vi "Mouse Up on Plot.vi"(7 "Loop data in":T1={"TitleCollapse"=refnum, "MouseDownState"=enum."Idle", "RightClickCache"={"Mod"={"Ctrl"=FALSE, "Shift"=FALSE}, "CoordsStart"={"Horizontal"=0, "Vertical"=0}, "CoordsEnd"={"Horizontal"=0, "Vertical"=0}, "PlotAreaBounds"={"Left"=10, "Top"=10, "Right"=0, "Bottom"=0}, "slice"=[]}, "ZoomCache"={"SuppressedPlots"=[], "LeftAxis"={"NeedsRevert?"=FALSE, "Scale Fit"=0, "Range"={"Minimum"=0.0, "Maximum"=0.0, "Increment"=0.0, "Minor Increment"=0.0, "Start"=0.0}}, "RightAxis"={"NeedsRevert?"=FALSE, "Scale Fit"=0, "Range"={"Minimum"=0.0, "Maximum"=0.0, "Increment"=0.0, "Minor Increment"=0.0, "Start"=0.0}}, "Mod"={"Shift"=FALSE}}, "UpdateTime"=0.0, "keyboard"=refnum, "visible?"=FALSE}, 8 "error in (no error)":errorcluster, 11 "Refs":T12) -> (0 "error out":errorcluster, 5 "Loop data out":T1={"TitleCollapse"=refnum, "MouseDownState"=enum."Idle", "RightClickCache"={"Mod"={"Ctrl"=FALSE, "Shift"=FALSE}, "CoordsStart"={"Horizontal"=0, "Vertical"=0}, "CoordsEnd"={"Horizontal"=0, "Vertical"=0}, "PlotAreaBounds"={"Left"=10, "Top"=10, "Right"=0, "Bottom"=0}, "slice"=[]}, "ZoomCache"={"SuppressedPlots"=[], "LeftAxis"={"NeedsRevert?"=FALSE, "Scale Fit"=0, "Range"={"Minimum"=0.0, "Maximum"=0.0, "Increment"=0.0, "Minor Increment"=0.0, "Start"=0.0}}, "RightAxis"={"NeedsRevert?"=FALSE, "Scale Fit"=0, "Range"={"Minimum"=0.0, "Maximum"=0.0, "Increment"=0.0, "Minor Increment"=0.0, "Start"=0.0}}, "Mod"={"Shift"=FALSE}}, "UpdateTime"=0.0, "keyboard"=refnum, "visible?"=FALSE})   [LabVIEW 2021, in "RocketPlot.lvlib"]
uses:
  RocketPlot.lvlib
  TypeDefs/Plot UI references.ctl
  Classes/RocketPlotHandle/RocketPlotHandle.lvclass
  <userlib>/bjustice/TipStripOOPanel/Classes/TipPanelHandle/TipPanelHandle.lvclass
  TypeDefs/Plot top row.ctl
  TypeDefs/plot while loop data.ctl
  CollapsePanel/CollapsePanel.lvclass
  TypeDefs/MouseDownState.ctl
  TypeDefs/RightClickCache.ctl
  TypeDefs/RightClickCache PlatMod.ctl
  <vilib>/Utility/miscctls.llb/LVPoint32TypeDef.ctl
  <vilib>/Utility/miscctls.llb/LVRectTypeDef.ctl
  TypeDefs/Slice average.ctl
  TypeDefs/ZoomCache.ctl
  TypeDefs/RangeCache.ctl
  <vilib>/Utility/miscctls.llb/LVRangeTypeDef.ctl
  TypeDefs/ZoomCache PlatMod.ctl
  <userlib>/bjustice/TipStripOOPanel/Classes/TipPanelHandle/CMD - hide.vi
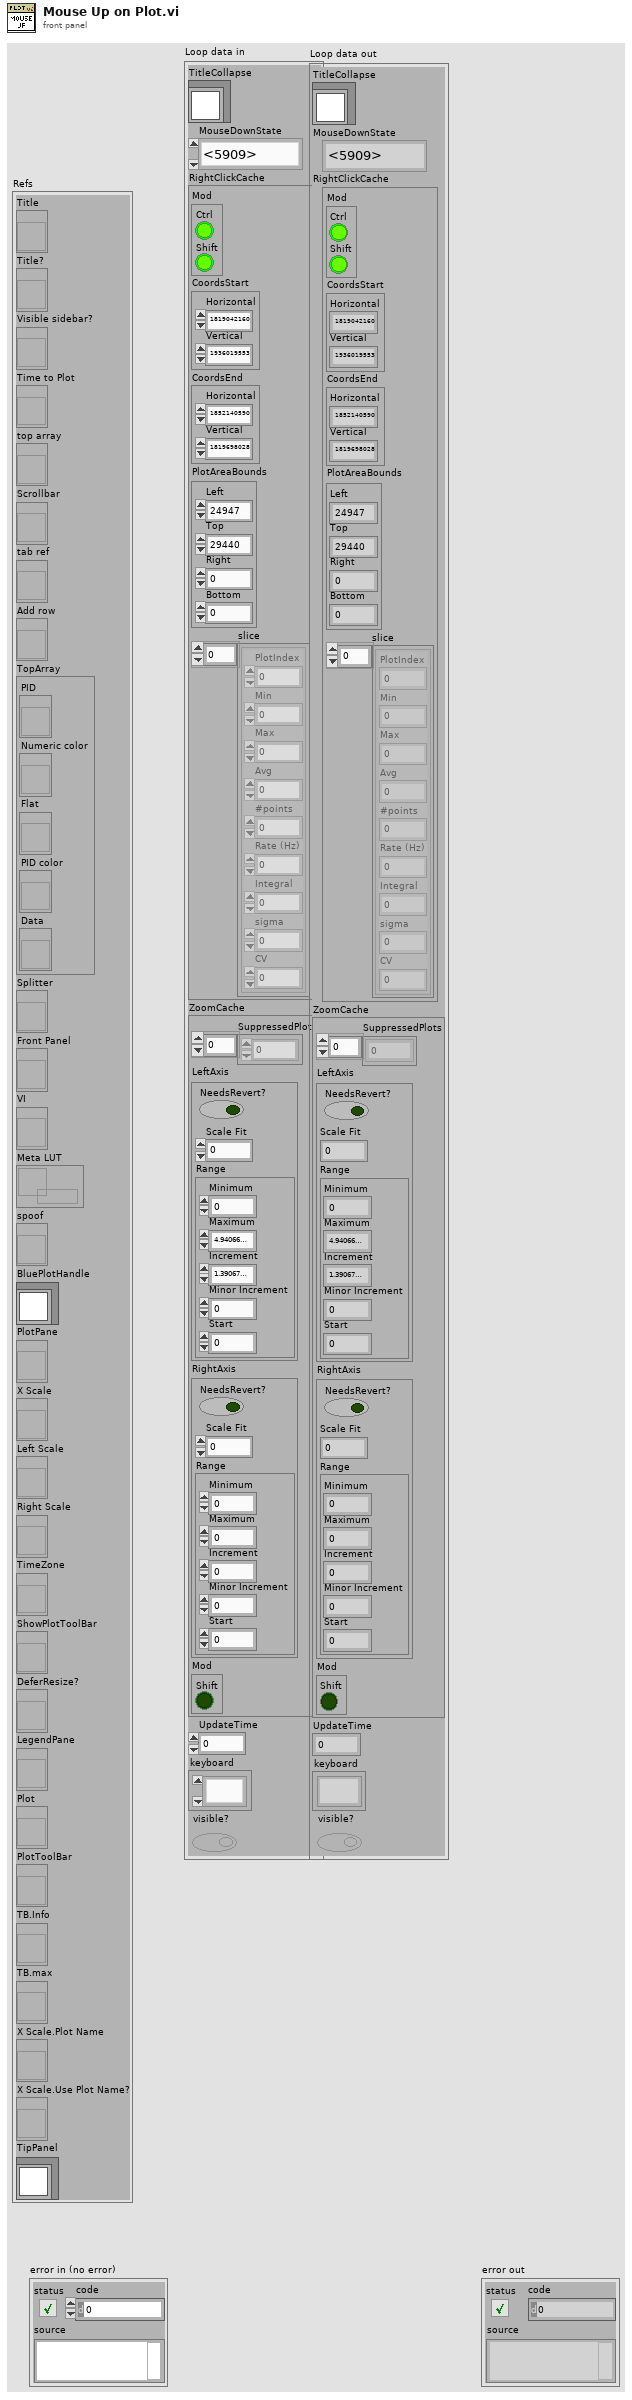
[diagram p1: front panel]
types:
  T1 = typedef "RocketPlot.lvlib/plot while loop data.ctl" = cluster{"TitleCollapse":refnum<class "CollapsePanel.lvclass">, "MouseDownState":T2, "RightClickCache":T3, "ZoomCache":T8, "UpdateTime":dbl, "keyboard":refnum<k1>, "visible?":bool}
  T2 = typedef "RocketPlot.lvlib/MouseDownState.ctl" = enum16{"Idle", "Pan", "Zoom", "Zoom-Post", "RightClick"}
  T3 = typedef "RocketPlot.lvlib/RightClickCache.ctl" = cluster{"Mod":T4, "CoordsStart":T5, "CoordsEnd":T5, "PlotAreaBounds":T6, "slice":T7[]}
  T4 = typedef "RocketPlot.lvlib/RightClickCache PlatMod.ctl" = cluster{"Ctrl":bool, "Shift":bool}
  T5 = typedef "LVPoint32TypeDef.ctl" = cluster{"Horizontal":i32, "Vertical":i32}
  T6 = typedef "LVRectTypeDef.ctl" = cluster{"Left":i16, "Top":i16, "Right":i16, "Bottom":i16}
  T7 = typedef "RocketPlot.lvlib/Slice average.ctl" = cluster{"PlotIndex":i32, "Min":dbl, "Max":dbl, "Avg":dbl, "#points":u32, "Rate (Hz)":dbl, "Integral":dbl, "sigma":dbl, "CV":dbl}
  T8 = typedef "RocketPlot.lvlib/ZoomCache.ctl" = cluster{"SuppressedPlots":i32[], "LeftAxis":T9, "RightAxis":T9, "Mod":T11}
  T9 = typedef "RocketPlot.lvlib/RangeCache.ctl" = cluster{"NeedsRevert?":bool, "Scale Fit":u8, "Range":T10}
  T10 = typedef "LVRangeTypeDef.ctl" = cluster{"Minimum":dbl, "Maximum":dbl, "Increment":dbl, "Minor Increment":dbl, "Start":dbl}
  T11 = typedef "RocketPlot.lvlib/ZoomCache PlatMod.ctl" = cluster{"Shift":bool}
  T12 = typedef "RocketPlot.lvlib/Plot UI references.ctl" = cluster{"Title":refnum<vi>, "Title?":refnum<vi>, "Visible sidebar?":refnum<vi>, "Time to Plot":refnum<vi>, "top array":refnum<vi>, "Scrollbar":refnum<vi>, "tab ref":refnum<vi>, "Add row":refnum<vi>, "TopArray":cluster{"PID":refnum<vi>, "Numeric color":refnum<vi>, "Flat":refnum<vi>, "PID color":refnum<vi>, "Data":refnum<vi>}, "Splitter":refnum<vi>, "Front Panel":refnum<vi>, "VI":refnum<vi>, "Meta LUT":refnum<data-value>, "spoof":refnum<vi>, "BluePlotHandle":refnum<class "RocketPlotHandle.lvclass">, "PlotPane":refnum<vi>, "X Scale":refnum<vi>, "Left Scale":refnum<vi>, "Right Scale":refnum<vi>, "TimeZone":refnum<vi>, "ShowPlotToolBar":refnum<vi>, "DeferResize?":refnum<vi>, "LegendPane":refnum<vi>, "Plot":refnum<vi>, "PlotToolBar":refnum<vi>, "TB.Info":refnum<vi>, "TB.max":refnum<vi>, "X Scale.Plot Name":refnum<vi>, "X Scale.Use Plot Name?":refnum<vi>, "TipPanel":refnum<class "TipPanelHandle.lvclass">}
  T13 = cluster{"Left":i32, "Top":i32, "Right":i32, "Bottom":i32}
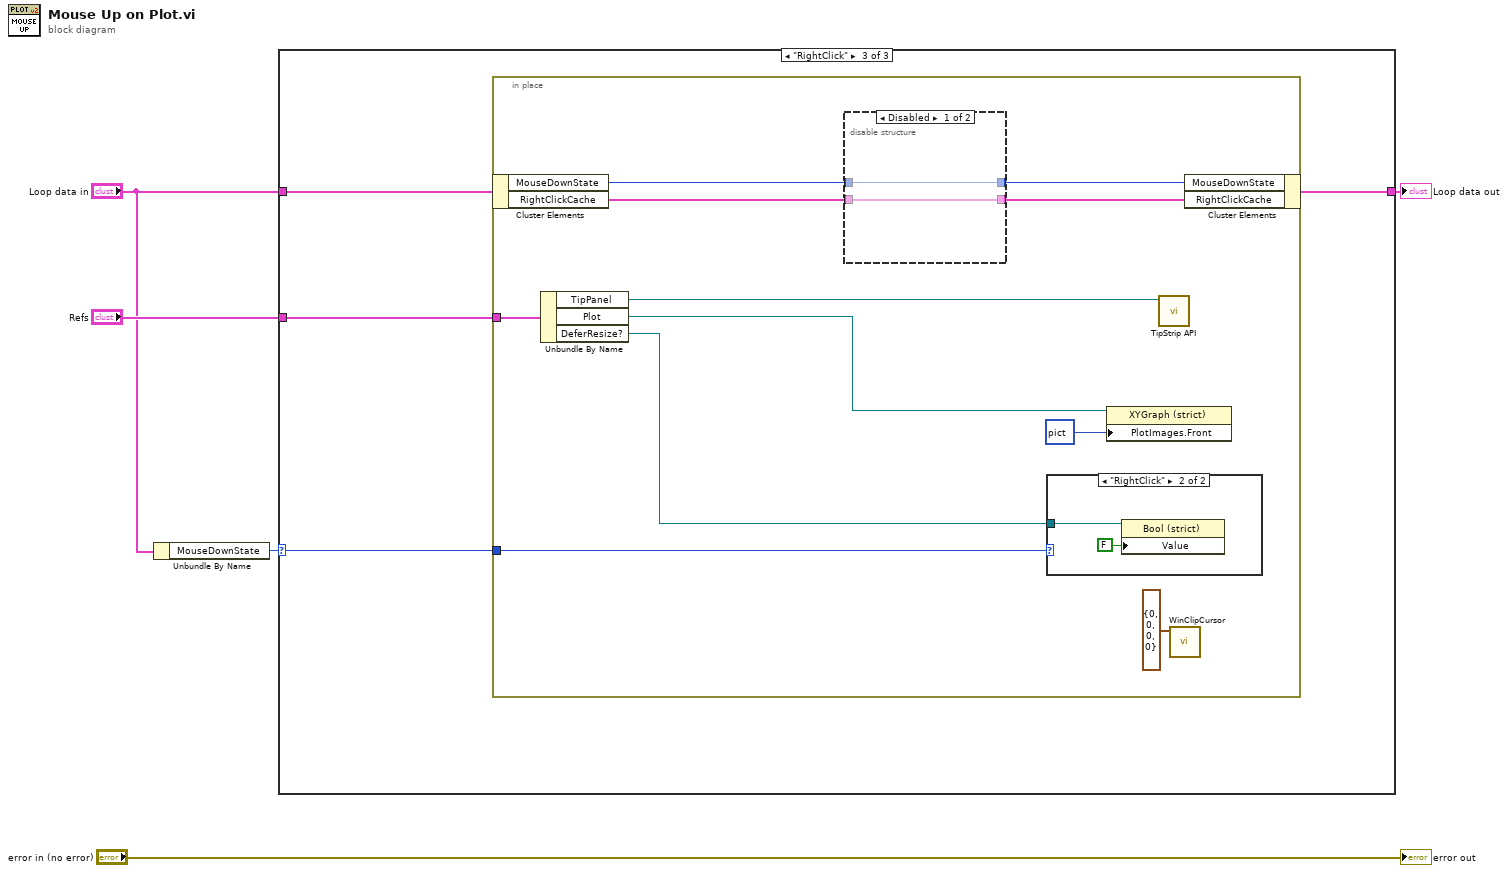
[diagram p0: block diagram]
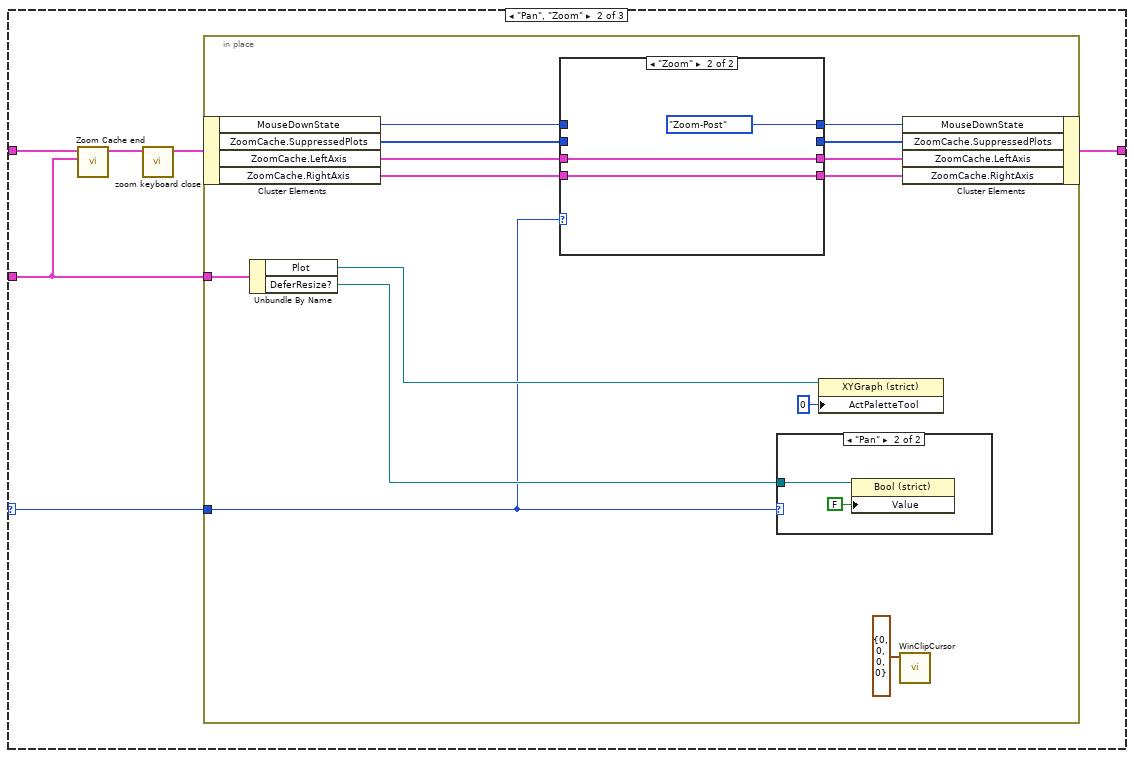
[diagram p3: hidden frame]
diagram:
  n1 = Unbundle By Name("Loop data in") -> ("MouseDownState"=w5:T2)
  n2 = case shown="\"RightClick\"" w5 {
    selector: w5 -> [_ w11 w44]
    tunnel: "Refs" -> [_ w9 w46]
    tunnel: "Loop data in" -> [w6 w10 w47]
    tunnel: [w6 w12 w45] -> w2
    frame "Idle", "Zoom-Post" {
    }
    frame "Pan", "Zoom" {
      n3 = call "Zoom Cache end.vi"("Refs"=w9, "Loop data in"=w10) -> ("Loop data out"=w8:T1)  [unwired: 8 in, 1 out]
      n4 = call "zoom keyboard close.vi"("Loop data in"=w8) -> ("Loop data out"=w7:T1)  [unwired: 9 in, 1 out]
      n5 = in-place {
        in-place-border: w9 -> [w26]
        in-place-border: w11 -> [w22]
        n6 = in-place-cluster #1(w7) -> ("MouseDownState"=w20:T2, "ZoomCache.SuppressedPlots"=w19:i32[], "ZoomCache.LeftAxis"=w17:T9, "ZoomCache.RightAxis"=w15:T9)
        n7 = Unbundle By Name(w26) -> ("Plot"=w25:refnum<vi>, "DeferResize?"=w24:refnum<vi>)
        n8 = case shown="\"Zoom\"" w22 {
          tunnel: w20 -> [w34 _]
          tunnel: [w30 MouseDownState."Zoom-Post" ("ScaleState")] -> w21
          tunnel: w19 -> [w33 _]
          tunnel: [w29 _] -> w18
          tunnel: w17 -> [w32 w40]
          tunnel: [w28 w40] -> w16
          tunnel: w15 -> [w31 w39]
          tunnel: [w27 w39] -> w14
          frame Default {
            n9 = disable-structure shown="Enabled" {
              disable-tunnel: [w38 _] -> w29
              disable-tunnel: w33 -> [w38 _]
              disable-tunnel: w32 -> [w37 _]
              disable-tunnel: [w37 _] -> w28
              disable-tunnel: [w36 _] -> w27
              disable-tunnel: w31 -> [w36 _]
              disable-tunnel: [w35 _] -> w30
              disable-tunnel: w34 -> [w35 _]
              frame Disabled {
              }
              frame Enabled {
              }
            }
          }
          frame "Zoom" {
          }
        }
        n10 = case shown="\"Pan\"" w22 {
          tunnel: w24 -> [_ w43]
          frame Default {
          }
          frame "Pan" {
            n11 = property class="Bool (strict)"(reference=w43, "Value"=FALSE) -> ()  [unwired: 1 in, 2 out]
          }
        }
        n12 = property class="XYGraph (strict)"(reference=w25, "ActPaletteTool"=0 ("Palette:Active Tool")) -> ()  [unwired: 1 in, 2 out]
        n13 = call "WinClipCursor.vi"("RECT"=T13 {"Left"=0, "Top"=0, "Right"=0, "Bottom"=0}) -> ()  [unwired: 10 in, 1 out]
        n14 = in-place-cluster #1("MouseDownState"=w21, "ZoomCache.SuppressedPlots"=w18, "ZoomCache.LeftAxis"=w16, "ZoomCache.RightAxis"=w14) -> (w12:T1)
      }
    }
    frame "RightClick" {
      n15 = in-place {
        in-place-border: w46 -> [w58]
        in-place-border: w44 -> [w56]
        n16 = in-place-cluster #2(w47) -> ("MouseDownState"=w52:T2, "RightClickCache"=w49:T3)
        n17 = Unbundle By Name(w58) -> ("TipPanel"=w48:refnum<class "TipPanelHandle.lvclass">, "Plot"=w54:refnum<vi>, "DeferResize?"=w57:refnum<vi>)
        n18 = disable-structure shown="Disabled" {
          disable-tunnel: w52 -> [w60 _]
          disable-tunnel: [w60 _] -> w51
          disable-tunnel: [w59 _] -> w50
          disable-tunnel: w49 -> [w59 _]
          frame Disabled {
          }
          frame Enabled {
          }
        }
        n19 = case shown="\"RightClick\"" w56 {
          tunnel: w57 -> [_ w62]
          frame Default {
          }
          frame "RightClick" {
            n20 = property class="Bool (strict)"(reference=w62, "Value"=FALSE) -> ()  [unwired: 1 in, 2 out]
          }
        }
        n21 = property class="XYGraph (strict)"(reference=w54, "PlotImages.Front"=picture data[5B] ("Plot Images:Front")) -> ()  [unwired: 1 in, 2 out]
        n22 = call-poly <userlib>:"TipStrip API.vi"("TipPanelHandle"=w48) -> ()  [unwired: 9 in, 2 out]
        n23 = call "WinClipCursor.vi"("RECT"=T13 {"Left"=0, "Top"=0, "Right"=0, "Bottom"=0}) -> ()  [unwired: 10 in, 1 out]
        n24 = in-place-cluster #2("MouseDownState"=w51, "RightClickCache"=w50) -> (w45:T1)
      }
    }
  }
  "Loop data out" <- w2
  "error out" <- "error in (no error)"
